vi "Exit.vi"(8 "error in (no error)":errorcluster, 11 "Old State":refnum<class "State Actor.lvclass">) -> (0 "error out":errorcluster, 3 "New State":refnum<class "State Actor.lvclass">)   [LabVIEW 2014, in "Robot Actors.lvlib" / "State Actor.lvclass"]
doc: "This is an abstract method. Override this method to define the behavior when you leave the state."
uses:
  State Actor.lvclass
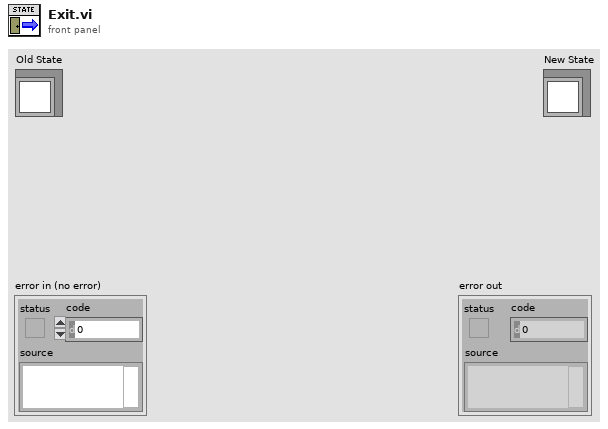
[diagram p1: front panel]
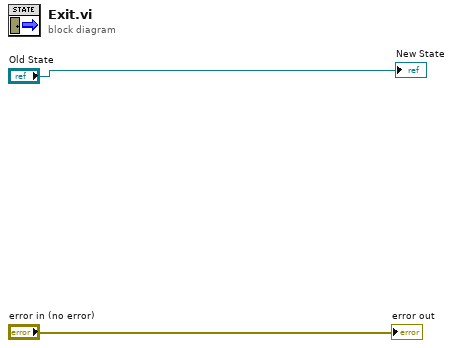
[diagram p0: block diagram]
diagram:
  "error out" <- "error in (no error)"
  "New State" <- "Old State"
